vi "test Get-Set-Get Hardware Configuration File.vi"(8 "error in":errorcluster, 11 "TestCase in":refnum<class "Scripting.lvclass">=refnum) -> (0 "error out":errorcluster, 3 "TestCase out":refnum<class "Scripting.lvclass">)   [LabVIEW 2020, in "Scripting.lvclass"]
uses:
  Scripting.lvclass
  <vilib>/addons/_JKI Toolkits/VI Tester/TestCase.llb/TestCase.lvclass
  Scripting/AIM MIL-STD-1553 Scripting.lvlib
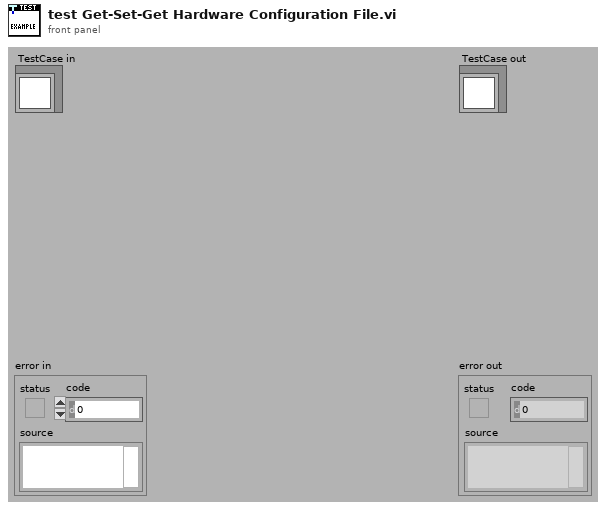
[diagram p1: front panel]
types:
  T1 = typedef "Custom Device API.lvlib/Custom Device Item Ref.ctl" = u64
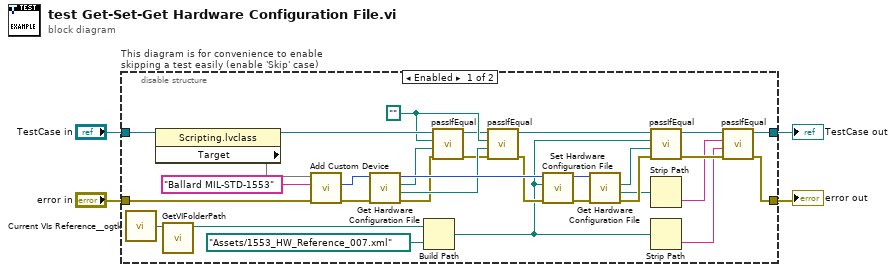
[diagram p0: block diagram]
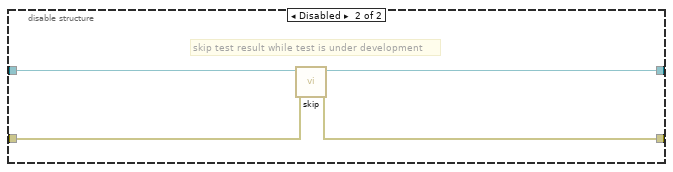
[diagram p2: hidden frame]
diagram:
  n1 = disable-structure "This diagram is for convenience to enable skipping a test easily (enable 'Skip' case)" shown="Enabled" {
    disable-tunnel: "TestCase in" -> [w33 w39]
    disable-tunnel: [w8 w37] -> w1
    disable-tunnel: [w7 w38] -> w3
    disable-tunnel: "error in" -> [w35 w36]
    frame Enabled {
      w21 = path ""
      n2 = call <userlib>:"Current VIs Reference__ogtk.vi"() -> ("Current VI's reference"=w26:refnum<vi>)  [unwired: 5 in]
      n3 = property class="Scripting.lvclass"(reference=w33) -> (reference out=w31:refnum<class "Scripting.lvclass">, "Target"=w32)  [unwired: 1 in, 1 out]
      n4 = call "GetVIFolderPath.vi"("VI Reference in"=w26) -> ("VI Folder Path out"=w27:path)  [unwired: 9 in, 1 out]
      n5 = call "Add Custom Device.vi"("error in"=w35, "name"="Ballard MIL-STD-1553", "target in"=w32) -> ("error out"=w29:errorcluster, "Ballard MIL-STD 1553 custom device"=w30:T1)  [unwired: 6 in, 1 out]
      n6 = call "Get Hardware Configuration File.vi"("error in"=w29, "Ballard MIL-STD 1553 custom device in"=w30) -> ("error out"=w19:errorcluster, "RT destination"=w20:path, "hardware configuration file"=w22:path, "Ballard MIL_STD 1553 custom device out"=w24:T1)  [unwired: 6 in]
      n7 = Build Path(base path=w27, name or relative path=path "Assets/1553_HW_Reference_007.xml" ("hardware configuration file path")) -> (appended path=w5:path)
      n8 = call-dynamic "passIfEqual.vi"("error in (no error)"=w19, "y"=w22, "x"=w21, "TestCase in"=w31) -> ("error out"=w17:errorcluster, "TestCase out"=w18:refnum<class "Scripting.lvclass">)  [unwired: 6 in]
      n9 = call-dynamic "passIfEqual.vi"("error in (no error)"=w17, "y"=w20, "x"=w21, "TestCase in"=w18) -> ("error out"=w16:errorcluster, "TestCase out"=w15:refnum<class "Scripting.lvclass">)  [unwired: 6 in]
      n10 = call "Set Hardware Configuration File.vi"("error in"=w16, "hardware configuration file path"=w5, "Ballard MIL-STD 1553 custom device in"=w24) -> ("error out"=w28:errorcluster, "Ballard MIL-STD 1553 custom device out"=w23:T1)  [unwired: 7 in]
      n11 = call "Get Hardware Configuration File.vi"("error in"=w28, "Ballard MIL-STD 1553 custom device in"=w23) -> ("error out"=w14:errorcluster, "RT destination"=w13:path, "hardware configuration file"=w6:path)  [unwired: 6 in, 1 out]
      n12 = call-dynamic "passIfEqual.vi"("error in (no error)"=w14, "y"=w6, "x"=w5, "TestCase in"=w15) -> ("error out"=w12:errorcluster, "TestCase out"=w9:refnum<class "Scripting.lvclass">)  [unwired: 6 in]
      n13 = Strip Path(path=w13) -> (name=w11:string)  [unwired: 1 out]
      n14 = Strip Path(path=w5) -> (name=w10:string)  [unwired: 1 out]
      n15 = call-dynamic "passIfEqual.vi"("error in (no error)"=w12, "y"=w10, "x"=w11, "TestCase in"=w9) -> ("error out"=w7:errorcluster, "TestCase out"=w8:refnum<class "Scripting.lvclass">)  [unwired: 6 in]
    }
    frame Disabled {
      # "skip test result while test is under development"
      n16 = call <vilib>:"skip.vi"("error in (no error)"=w36, "TestCase in"=w39) -> ("error out"=w38:errorcluster, "TestCase out"=w37:refnum<class "TestCase.lvclass">)  [unwired: 8 in]
    }
  }
  "error out" <- w3
  "TestCase out" <- w1
